vi "Actor Core.vi"(8 "error in":errorcluster, 11 "Cooler UI":refnum<class "Live User Controller.lvclass">) -> (0 "error out":errorcluster, 3 "Actor out":refnum<class "Actor.lvclass">)   [LabVIEW 2025, in "Live User Controller.lvclass"]
doc: "This is Actor Core.vi, the main message handling loop for Actors. An actor usually just sits in this loop and processes messages as they arrive. Any error returned by the message Do.vi call will stop the loop, with error code 43 as the canonical signal to stop with no error sent to caller. Descendants may override that in Handle Error.vi."
uses:
  Live User Controller.lvclass
  C:/Program Files/National Instruments/LabVIEW 2025/vi.lib/ActorFramework/Actor/Actor.lvclass
  C:/Program Files/National Instruments/LabVIEW 2025/ProjectTemplates/Source/Core/Feedback Evaporative Cooler/Cooler Controller/Cooler Controller/Cooler Controller.lvclass
  <vilib>/ActorFramework/Actor/Actor.lvclass
  <vilib>/ActorFramework/Actor/Actor.lvclass/Actor.ctl
  Cooler Controller/Cooler Controller/Cooler Controller.lvclass/Cooler Controller.ctl
  <vilib>/ActorFramework/Message Enqueuer/Message Enqueuer.lvclass/Message Enqueuer.ctl
  Air Cooler Application/Load Into Sub Panel Msg/Load Into Sub Panel Msg.lvclass/Load Into Sub Panel Msg.ctl
  Cooler Controller/Change Desired Temperature Msg/Change Desired Temperature Msg.lvclass/Change Desired Temperature Msg.ctl
  <vilib>/ActorFramework/Stop Msg/Stop Msg.lvclass/Stop Msg.ctl
  <vilib>/ActorFramework/Message Enqueuer/Init from Existing Queue.vi
  <vilib>/ActorFramework/Message Enqueuer/Enqueue.vi
  <vilib>/ActorFramework/Message Enqueuer/Enqueue Critical.vi
  Cooler Controller/Change Desired Temperature Msg/Change Desired Temperature Msg.lvclass
  C:/Program Files/National Instruments/LabVIEW 2025/vi.lib/ActorFramework/Message/Message.lvclass
  <vilib>/ActorFramework/Stop Msg/Stop Msg.lvclass
  Air Cooler Application/Load Into Sub Panel Msg/Load Into Sub Panel Msg.lvclass
  <vilib>/ActorFramework/Message Priority Queue/Priority Enqueue.vi
  <vilib>/ActorFramework/Message Enqueuer/Message Enqueuer.lvclass
  Evaporative Cooler Controller/Evaporative Cooler Controller/Evaporative Cooler Controller.lvclass
  Cooler Controller/Cooler Controller/Cooler Controller.lvclass
panel:
  in  "stop":bool
  out "Water Pump Active?":dbl(slide) scale=0.0..25.0
  out "Fault B":bool caption="Fault Detected"
  in  "Desired Temperature":dbl=75.0
  out "Actual Temperature":dbl(slide) scale=60.0..120.0
  out "Fault A":bool caption="Fault Detected"
  out "Fan B":bool
  out "Fan A":bool
  out "Water Basin":dbl(slide)=10.459183673469388 scale=0.0..25.0
  out "Pump Status":bool
  # "Fans spin up 5 seconds after water pump starts."
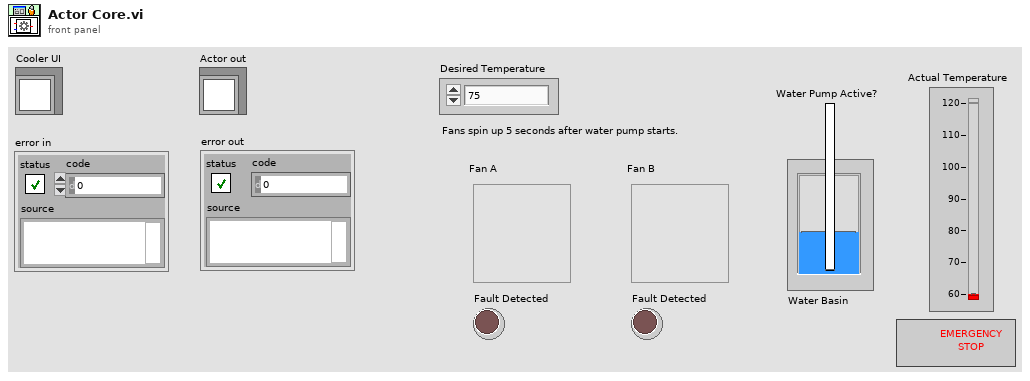
[diagram p1: front panel]
types:
  T1 = cluster{"Pump Status":bool, "Pump Level":dbl, "Pump Dir":bool}
  T2 = cluster{"Actual Temperature":refnum<vi>, "Fan A":refnum<vi>, "Fault A":refnum<vi>, "Fan B":refnum<vi>, "Fault B":refnum<vi>, "Pump Status":refnum<vi>, "Water Basin":refnum<vi>}
  T3 = enum32{"Invalid", "Standard", "Closed", "Hidden", "Minimized", "Maximized"}
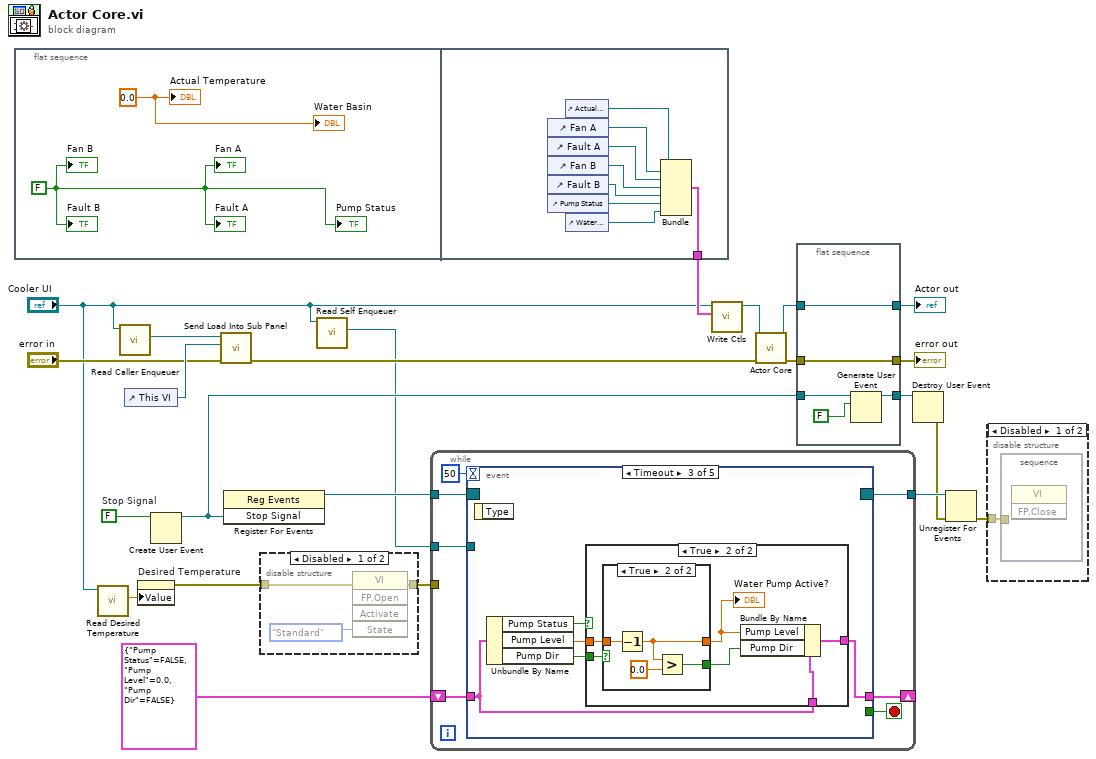
[diagram p0: block diagram]
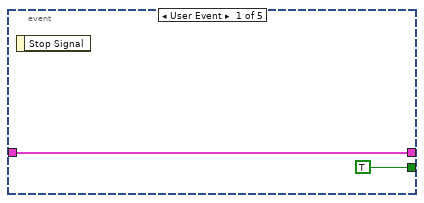
[diagram p4: hidden frame]
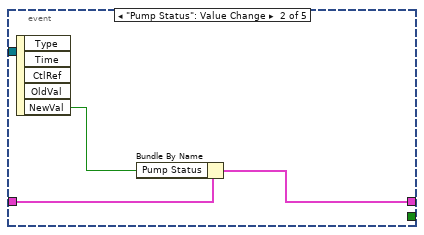
[diagram p5: hidden frame]
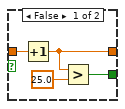
[diagram p7: hidden frame]
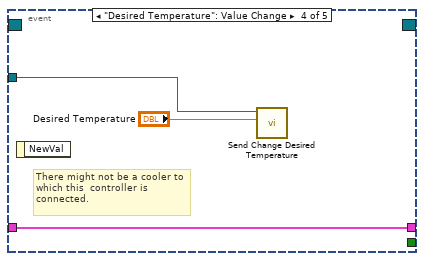
[diagram p8: hidden frame]
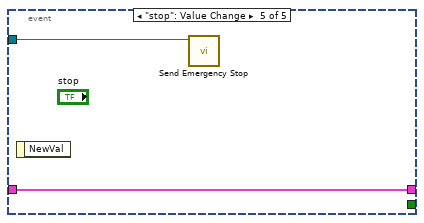
[diagram p9: hidden frame]
diagram:
  w20 = FALSE  # Stop Signal
  n1 = flat-sequence {
    tunnel: [w28] -> w22
    frame #0 {
      w24 = 0.0 ("value")
      w25 = FALSE
      "Actual Temperature" <- w24
      "Fan A" <- w25
      "Fan B" <- w25
      "Fault A" <- w25
      "Fault B" <- w25
      "Pump Status" <- w25
      "Water Basin" <- w24
    }
    frame #1 {
      n2 = control-ref of="Fan A"() -> (w30:refnum<vi>)
      n3 = control-ref of="Fault A"() -> (w31:refnum<vi>)
      n4 = control-ref of="Fan B"() -> (w29:refnum<vi>)
      n5 = control-ref of="Fault B"() -> (w32:refnum<vi>)
      n6 = control-ref of="Pump Status"() -> (w27:refnum<vi>)
      n7 = control-ref of="Actual Temperature"() -> (w33:refnum<vi>)
      n8 = control-ref of="Water Basin"() -> (w26:refnum<vi>)
      n9 = Bundle("Actual Temperature"=w33, "Fan A"=w30, "Fault A"=w31, "Fan B"=w29, "Fault B"=w32, "Pump Status"=w27, "Water Basin"=w26) -> (w28:T2)  [unwired: 1 in]
    }
  }
  n10 = call "Read Desired Temperature.vi"("Cooler Controller in"="Cooler UI") -> ("Desired Temperature"=w7:dbl)  [unwired: 10 in]
  n11 = call <vilib>:"Read Caller Enqueuer.vi"("Actor"="Cooler UI") -> ("Caller Enqueuer"=w6:refnum<class "Message Enqueuer.lvclass">)  [unwired: 10 in]
  n12 = control-ref of="This VI"() -> (w5:refnum<vi>)
  n13 = property on="Desired Temperature" class="DigNum (strict)"("Value"=w7) -> (error out=w8:errorcluster)  [unwired: 2 in, 1 out]
  n14 = Create User Event(user event datatype=w20) -> (user event=w16:refnum<user-event>)  [unwired: 1 in, 1 out]
  n15 = call "Send Load Into Sub Panel.vi"("error in (no error)"="error in", "VI for SubPanel"=w5, "Message Enqueuer"=w6) -> ("error out"=w3:errorcluster)  [unwired: 8 in]
  n16 = register-events(w16) -> (reference out=w21:refnum<event-registration>)  [unwired: 2 in, 1 out]
  n17 = disable-structure shown="Disabled" {
    disable-tunnel: [w35 _] -> w10
    disable-tunnel: w8 -> [w34 _]
    frame Disabled {
      n18 = invoke class="VI" method="FP.Open"(error in=w34, "State"=T3."Standard") -> (error out=w35:errorcluster)  [unwired: 3 in, 4 out]
    }
    frame Enabled {
    }
  }
  n19 = call <vilib>:"Read Self Enqueuer.vi"("Actor"="Cooler UI") -> ("Self Enqueuer"=w1:refnum<class "Message Enqueuer.lvclass">)  [unwired: 10 in]
  n20 = while {
    tunnel: w21 -> [w43]
    tunnel: [w42] -> w19
    shift-right: [w40] -> _
    shift-left: T1 {"Pump Status"=FALSE, "Pump Level"=0.0, "Pump Dir"=FALSE} -> [w39]
    tunnel: w10 -> [_]
    tunnel: w1 -> [w37]
    stop <- w41 stop-if-true
    n21 = event shown="[2] Timeout" {
      selector: w43 -> [_ _ _ _ _]
      dyn-events: [_ _ _ _ _] -> w42
      timeout: 50 -> [_ _ _ _ _]
      tunnel: [TRUE _ _ _ _] -> w41
      tunnel: [w44 w47 w51 w71 w73] -> w40
      tunnel: w39 -> [w44 w48 w50 w71 w73]
      tunnel: w37 -> [_ _ _ w70 w72]
      event User Event {
        n22 = event-data() -> ()  [unwired: 1 in, 1 out]
      }
      event "Pump Status": Value Change {
        n23 = event-data() -> ("NewVal"=w46:bool)  [unwired: 1 in, 4 out]
        n24 = Bundle By Name(cluster=w48, "Pump Status"=w46) -> (w47:T1)
      }
      event Timeout {
        n25 = event-data() -> ()  [unwired: 1 in, 1 out]
        n26 = Unbundle By Name(w50) -> ("Pump Status"=w53:bool, "Pump Level"=w49:dbl, "Pump Dir"=w52:bool)
        n27 = case shown="True" w53 {
          tunnel: w52 -> [_ w60]
          tunnel: [w54 w59] -> w51
          tunnel: w50 -> [w54 w58]
          tunnel: w49 -> [_ w57]
          frame False {
          }
          frame True {
            n28 = case shown="True" w60 {
              tunnel: w57 -> [w64 w68]
              tunnel: [w63 w67] -> w55
              tunnel: [w61 w65] -> w56
              frame False {
                n29 = Increment(x=w64) -> (x+1=w63:dbl)
                n30 = Greater?(x=w63, y=25.0) -> (0:w61:bool)
              }
              frame True {
                n31 = Decrement(x=w68) -> (x-1=w67:dbl)
                n32 = Greater?(x=w67, y=0.0) -> (0:w65:bool)
              }
            }
            "Water Pump Active?" <- w55
            n33 = Bundle By Name(cluster=w58, "Pump Level"=w55, "Pump Dir"=w56) -> (w59:T1)
          }
        }
      }
      event "Desired Temperature": Value Change {
        # "There might not be a cooler to which this  controller is connected."
        n34 = event-data() -> ()  [unwired: 1 in, 1 out]
        n35 = call "Send Change Desired Temperature.vi"("Desired Temperature"="Desired Temperature", "Message Enqueuer"=w70) -> ()  [unwired: 9 in, 1 out]
      }
      event "stop": Value Change {
        n36 = event-data() -> ()  [unwired: 1 in, 1 out]
        n37 = call <vilib>:"Send Emergency Stop.vi"("Message Enqueuer"=w72) -> ()  [unwired: 10 in, 1 out]
      }
    }
  }
  n38 = call "Write Ctls.vi"("Ctls"=w22, "Cooler UI in"="Cooler UI") -> ("Cooler UI out"=w23:refnum<class "Live User Controller.lvclass">)  [unwired: 9 in]
  n39 = call-parent "Actor Core.vi"("error in"=w3, "Actor in"=w23) -> ("error out"=w12:errorcluster, "Actor out"=w14:refnum<class "Actor.lvclass">)  [unwired: 8 in]
  n40 = flat-sequence {
    tunnel: [w78] -> w17
    tunnel: w16 -> [w77]
    tunnel: w14 -> [w76]
    tunnel: [w76] -> w15
    tunnel: w12 -> [w75]
    tunnel: [w75] -> w13
    frame #0 {
      n41 = Generate User Event(user event=w77, event data cluster=FALSE ("Stop Signal")) -> (user event out=w78:refnum<user-event>)  [unwired: 2 in, 1 out]
    }
  }
  n42 = Destroy User Event(user event=w17) -> (error out=w18:errorcluster)  [unwired: 1 in]
  n43 = Unregister For Events(event registration refnum=w19, error in=w18) -> (error out=w9:errorcluster)
  n44 = disable-structure shown="Disabled" {
    disable-tunnel: w9 -> [w79 _]
    frame Disabled {
      n45 = stacked-sequence {
        tunnel: w79 -> [_]
        frame #0 {
          n46 = invoke class="VI" method="FP.Close"() -> ()  [unwired: 3 in, 3 out]
        }
      }
    }
    frame Enabled {
    }
  }
  "error out" <- w13
  "Actor out" <- w15
